vi "RIOduino_COM.vi"() -> ()   [LabVIEW 2014]
uses:
  LED_Colors.ctl
  LED_Patterns.ctl
panel:
  in  "Pattern":T1=enum."Solid"
  in  "Color":T2
  in  "Section":u8
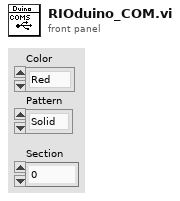
[diagram p1: front panel]
types:
  T1 = typedef "LED_Patterns.ctl" = enum8{"Black White", "Solid", "Blink", "Sweep", "Sleep"}
  T2 = typedef "LED_Colors.ctl" = enum8{"Red", "Green", "Blue", "Cyan", "Magenta", "Yellow"}
  T3 = typedef "WPI_I2CDevRef.ctl" = cluster{"DevStatus":errorcluster, "Controller":T4, "Device Address":u8, "Handle":i32, "I2C Bus":T5}
  T4 = typedef "FPGA_TypedefDigitalModule.ctl" = enum16{"Controller 1"}
  T5 = typedef "i2c_bus.ctl" = enum16{"I2C On-Board", "I2C MXP", "Invalid"}
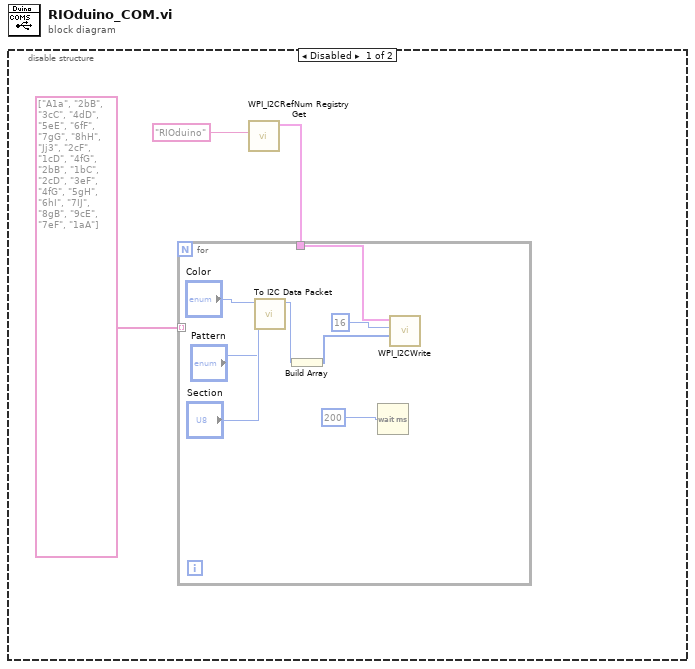
[diagram p0: block diagram]
diagram:
  n1 = disable-structure shown="Disabled" {
    frame Disabled {
      n2 = call <vilib>:"WPI_I2CRefNum Registry Get.vi"("refnum name"="RIOduino") -> ("I2CDevRef"=w2:T3)  [unwired: 9 in, 1 out]
      n3 = for {
        tunnel: w2 -> [w11]
        tunnel: string[] ["A1a", "2bB", "3cC", "4dD", "5eE", "6fF", "7gG", "8hH", "Jj3", "2cF", "1cD", "4fG", "2bB", "1bC", "2cD", "3eF", "4fG", "5gH", "6hI", "7IJ", "8gB", "9cE", "7eF", "1aA"] -> [_] mode=indexing
        n4 = call "To I2C Data Packet.vi"("Section"="Section", "Color"="Pattern", "Pattern"="Color") -> ("Output Byte"=w8:u8)  [unwired: 6 in, 2 out]
        n5 = Build Array(w8) -> (w6:u8[])
        n6 = Wait (ms)(milliseconds to wait=200) -> ()  [unwired: 1 out]
        n7 = call <vilib>:"WPI_I2CWrite.vi"("I2CDataToSend"=w6, "I2CRegister"=u8 16, "I2CDevRef"=w11) -> ()  [unwired: 7 in, 2 out]
      }
    }
    frame Enabled {
    }
  }
